vi "4Pi 4Pi Modes - Format Voltage Array.vi"(0 "Pixel Level (-1 to 1)":dbl[][](array[numeric])) -> (4 "Pixel Level (-1 to 1) Out":dbl[][](array[numeric]), 15 "Pixel Map":dbl[][][](array[numeric]))   [LabVIEW 2016]
uses:
  <vilib>/Analysis/baseanly.llb/Mean (DBL).vi
  <vilib>/Analysis/NI_AALBase.lvlib
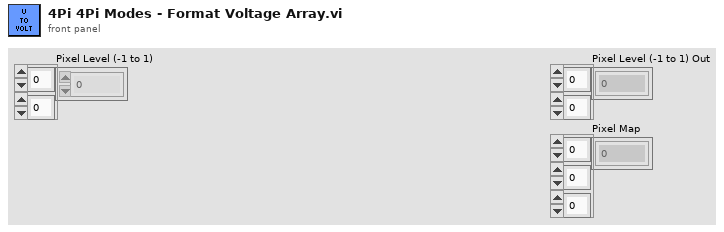
[diagram p1: front panel]
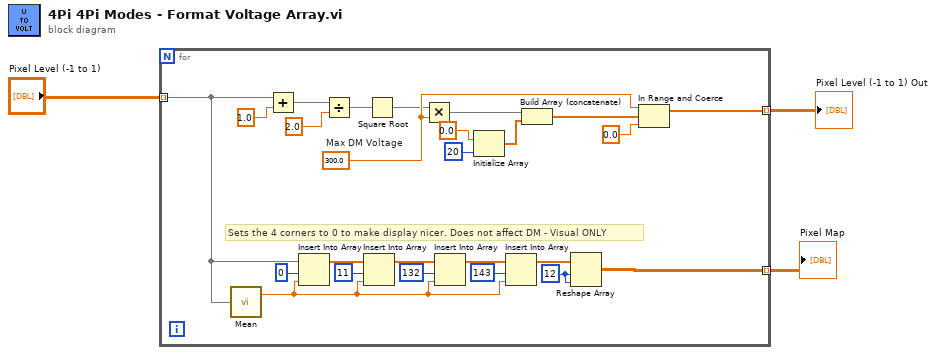
[diagram p0: block diagram]
diagram:
  n1 = for {
    tunnel: "Pixel Level (-1 to 1)" -> [w6] mode=indexing
    tunnel: [w5] -> w2 mode=indexing
    tunnel: [w4] -> w1 mode=indexing
    w28 = 300.0  # Max DM Voltage
    w14 = 12 ("dimension size")
    # "Sets the 4 corners to 0 to make display nicer. Does not affect DM - Visual ONLY"
    n2 = call-poly <vilib>:"Mean.vi"("X"=w6) -> ("mean"=w16:dbl)  [unwired: 1 out]
    n3 = Add(x=w6, y=1.0) -> (x+y=w21:dbl[])
    n4 = Insert Into Array(array=w6, index=0, new element=w16) -> (w9:dbl[])
    n5 = Divide(x=w21, y=2.0) -> (x/y=w23:dbl[])
    n6 = Insert Into Array(array=w9, index=11, new element=w16) -> (w11:dbl[])
    n7 = Square Root(x=w23) -> (sqrt(x)=w24:dbl[])
    n8 = Multiply(x=w24, y=w28) -> (x*y=w25:dbl[])
    n9 = Insert Into Array(array=w11, index=132, new element=w16) -> (w13:dbl[])
    n10 = Initialize Array(0.0 ("element"), 20 ("dimension size")) -> (w19:dbl[])
    n11 = Insert Into Array(array=w13, index=143, new element=w16) -> (w15:dbl[])
    n12 = Build Array (concatenate)(w25, w19) -> (w27:dbl[])
    n13 = Reshape Array(w15, w14, w14) -> (w4:dbl[][])
    n14 = In Range and Coerce(upper limit=w28, x=w27, lower limit=0.0) -> (coerced(x)=w5:dbl[])  [unwired: 1 out]
  }
  "Pixel Level (-1 to 1) Out" <- w2
  "Pixel Map" <- w1
